vi "Read COM.vi"(8 "error in (no error)":errorcluster, 11 "OHAUS_232 in":refnum<class "OHAUS_Navigator_232.lvclass">) -> (0 "error out":errorcluster, 2 "COM":refnum<visa-resource-name>, 3 "OHAUS_232 out":refnum<class "OHAUS_Navigator_232.lvclass">)   [LabVIEW 2019, in "OHAUS_Navigator_232.lvclass"]
uses:
  OHAUS_Navigator_232.lvclass
  OHAUS_Navigator_232.lvclass/OHAUS_Navigator_232.ctl
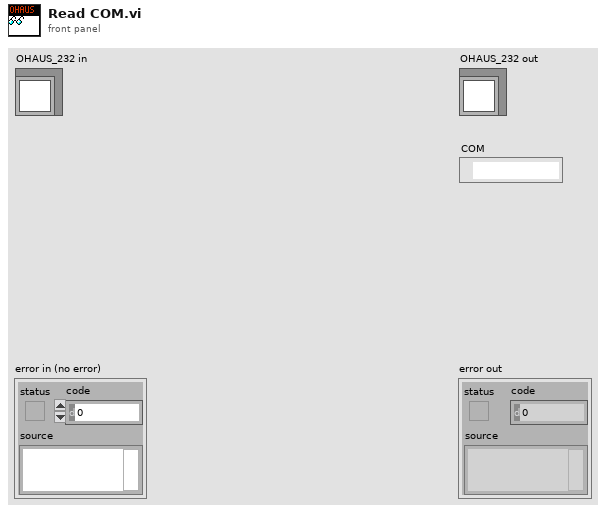
[diagram p1: front panel]
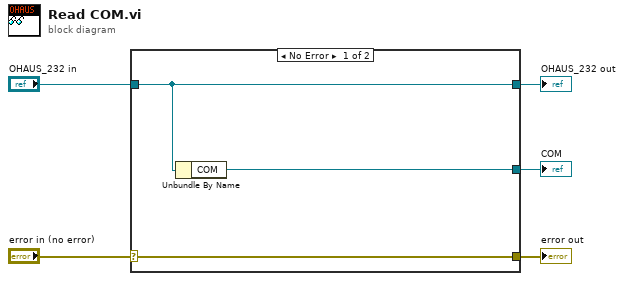
[diagram p0: block diagram]
diagram:
  n1 = case shown="No Error" "error in (no error)" {
    selector: "error in (no error)" -> [w8 w9]
    tunnel: [w8 w9] -> w4
    tunnel: [w7 w10] -> w2
    tunnel: "OHAUS_232 in" -> [w7 w10]
    tunnel: [w6 _] -> w1
    frame No Error {
      n2 = Unbundle By Name(w7) -> ("COM"=w6:refnum<visa-resource-name>)
    }
    frame Error {
    }
  }
  "error out" <- w4
  "OHAUS_232 out" <- w2
  "COM" <- w1
